vi "T7_Write_FLOAT32_Register.vi"(7 "FLOAT32 to Write":sgl=1.23, 9 "LabJack TestFLOAT32 Register":i32=55124, 10 "Remote Port":u16=502, 11 "Remote IP Address":string="192.168.1.15") -> ()   [LabVIEW 2014]
uses:
  Serial Link Layer/NI_Modbus_Cleaned/NI Modbus121Clean.llb/MB Ethernet Master Query Write Multiple Registers (poly).vi
panel:
  # "MB Ethernet Example Master.vi\n\nInstructions\n1.Use Kipling to find your devices IP address & modify the\n\"Remote IP Addres\"\n2. Run this VI\n3. Change value of \"FLOAT32 to Write\" & press \"Write Data\""
  # "TCP Parameters"
  # "Test Write & Read of TEST_UINT32 Register"
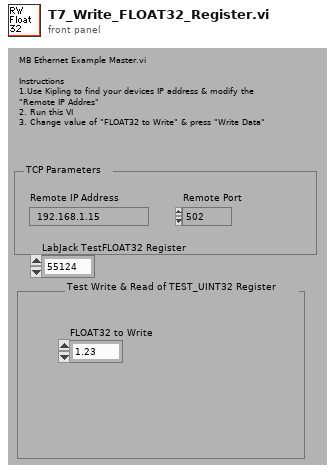
[diagram p1: front panel]
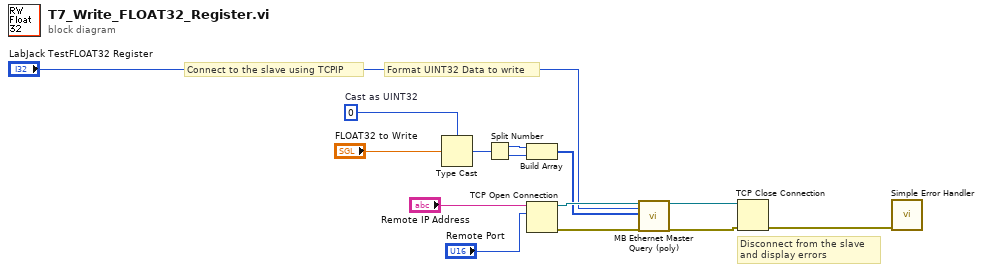
[diagram p0: block diagram]
diagram:
  w4 = u32 0  # Cast as UINT32
  # "Format UINT32 Data to write"
  # "Disconnect from the slave\nand display errors"
  # "Connect to the slave using TCPIP"
  n1 = Type Cast(type=w4, x="FLOAT32 to Write") -> (*(type *) &x=w3:u32)
  n2 = Split Number(x=w3) -> (hi(x)=w2:u16, lo(x)=w1:u16)
  n3 = Build Array(w2, w1) -> (w6:u16[])
  n4 = TCP Open Connection(address="Remote IP Address", remote port or service name="Remote Port") -> (connection ID=w12:refnum<k5>, error out=w11:errorcluster)  [unwired: 3 in]
  n5 = call-poly "MB Ethernet Master Query (poly).vi"("TCP Connection Refnum in"=w12, "Starting Address"="LabJack TestFLOAT32 Register", "Registers"=w6, "error in"=w11) -> ("TCP Connection Refnum (dup)"=w8:refnum<k5>, "error out"=w9:errorcluster)  [unwired: 13 in, 1 out]
  n6 = TCP Close Connection(connection ID=w8, error in (no error)=w9) -> (error out=w10:errorcluster)  [unwired: 2 out]
  n7 = call <vilib>:"Simple Error Handler.vi"("error in (no error)"=w10) -> ()  [unwired: 1 in, 8 out]
